vi "1D Buffer.vi"(1 "Data In":sgl[](array[numeric]), 2 "Reset":bool, 4 "buffer size":i32=1000) -> (0 "Buffer Out":sgl[](array[numeric]))   [LabVIEW 2014]
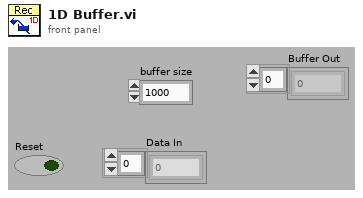
[diagram p1: front panel]
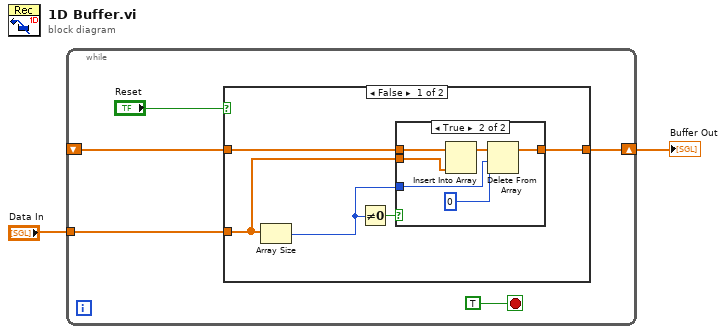
[diagram p0: block diagram]
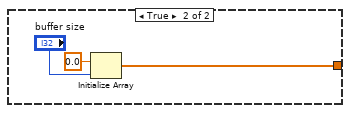
[diagram p3: hidden frame]
diagram:
  n1 = while {
    shift-right: [w4] -> w2
    shift-left: _ -> [w5]
    tunnel: "Data In" -> [w3]
    stop <- TRUE stop-if-true
    n2 = case shown="False" "Reset" {
      tunnel: [w11 w21] -> w4
      tunnel: w3 -> [w8 _]
      tunnel: w5 -> [w9 _]
      frame False {
        n3 = Array Size(array=w8) -> (size(s)=w10:i32)
        n4 = Not Equal To 0?(x=w10) -> (x != 0?=w12:bool)
        n5 = case shown="True" w12 {
          tunnel: w10 -> [_ w19]
          tunnel: [w13 w17] -> w11
          tunnel: w8 -> [_ w15]
          tunnel: w9 -> [w13 w16]
          frame False {
          }
          frame True {
            n6 = Insert Into Array(array=w16, new element=w15) -> (w14:sgl[])  [unwired: 1 in]
            n7 = Delete From Array(array=w14, length=w19, index=0 ("index (row)")) -> (array with subset deleted=w17:sgl[])  [unwired: 1 out]
          }
        }
      }
      frame True {
        n8 = Initialize Array(sgl 0.0 ("element"), "buffer size") -> (w21:sgl[])
      }
    }
  }
  "Buffer Out" <- w2
